vi "Clear Errors - Ext.vi"(8 "error in (no error)":errorcluster, 11 "specific error code to clear (0: all)":i32) -> (0 "error out":errorcluster)   [LabVIEW 2019]
doc: "<b>Description</b> This VI clears errors and can be used as an alternative to the stock Clear Errors VI. This VI is not not pull in any other library dependencies.\n\n<b>Inputs</b>\n<b>specific error code to clear</b>: Optionally specifies a specific error to clear.\n\n<b>Outputs</b>\n<b>error out</b>: Empty error if no specific error was specified or the specific error matches the input error.\n\nBSD 3-Clause License\n\nCopyright (c) 2021, TauTerra, LLC\nAll rights reserved.\n\nRedistribution and use in source and binary forms, with or without\nmodification, are permitted provided that the following conditions are met:\n\n1. Redistributions of source code must retain the above copyright notice, this\n list of conditions and the following disclaimer.\n\n2. Redistributions in binary form must reproduce the above copyright notice,\n this list of conditions and the following disclaimer in the documentation\n and/or other materials provided with the distribution.\n\n3. Neither the name of the copyright holder nor the names of its\n contributors may be used to endorse or promote products derived from\n this software without specific prior written permission.\n\nTHIS SOFTWARE IS PROVIDED BY THE COPYRIGHT HOLDERS AND CONTRIBUTORS \"AS IS\"\nAND ANY EXPRESS OR IMPLIED WARRANTIES, INCLUDING, BUT NOT LIMITED TO, THE\nIMPLIED WARRANTIES OF MERCHANTABILITY AND FITNESS FOR A PARTICULAR PURPOSE ARE\nDISCLAIMED. IN NO EVENT SHALL THE COPYRIGHT HOLDER OR CONTRIBUTORS BE LIABLE\nFOR ANY DIRECT, INDIRECT, INCIDENTAL, SPECIAL, EXEMPLARY, OR CONSEQUENTIAL\nDAMAGES (INCLUDING, BUT NOT LIMITED TO, PROCUREMENT OF SUBSTITUTE GOODS OR\nSERVICES; LOSS OF USE, DATA, OR PROFITS; OR BUSINESS INTERRUPTION) HOWEVER\nCAUSED AND ON ANY THEORY OF LIABILITY, WHETHER IN CONTRACT, STRICT LIABILITY,\nOR TORT (INCLUDING NEGLIGENCE OR OTHERWISE) ARISING IN ANY WAY OUT OF THE USE\nOF THIS SOFTWARE, EVEN IF ADVISED OF THE POSSIBILITY OF SUCH DAMAGE."
panel:
  out "specific error cleared?":bool
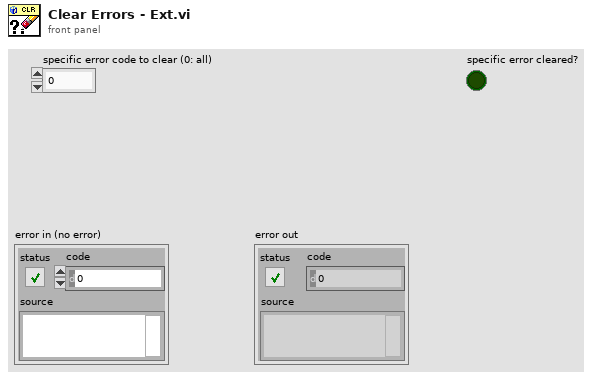
[diagram p1: front panel]
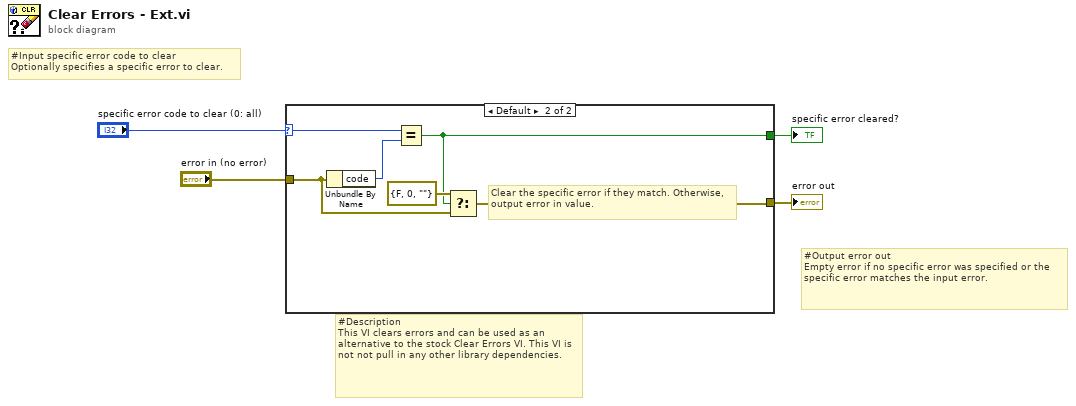
[diagram p0: block diagram]
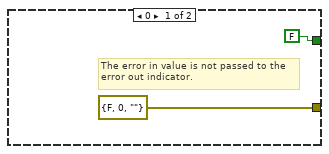
[diagram p2: hidden frame]
diagram:
  # "#Output error out\nEmpty error if no specific error was specified or the specific error matches the input error."
  # "#Input specific error code to clear\nOptionally specifies a specific error to clear."
  # "#Description\nThis VI clears errors and can be used as an alternative to the stock Clear Errors VI. This VI is not not pull in any other library dependencies."
  n1 = case shown="Default" "specific error code to clear (0: all)" {
    selector: "specific error code to clear (0: all)" -> [_ w11]
    tunnel: "error in (no error)" -> [_ w10]
    tunnel: [errorcluster {"status"=FALSE, "code"=0, "source"=""} ("error constant") w7] -> w1
    tunnel: [FALSE w8] -> w3
    frame 0 {
      # "The error in value is not passed to the\nerror out indicator."
    }
    frame Default {
      # "Clear the specific error if they match. Otherwise, output error in value."
      n2 = Unbundle By Name(w10) -> ("code"=w12:i32)
      n3 = Equal?(x=w11, y=w12) -> (x = y?=w8:bool)
      n4 = Select(t=errorcluster {"status"=FALSE, "code"=0, "source"=""} ("error constant"), s=w8, f=w10) -> (s? t:f=w7:errorcluster)
    }
  }
  "error out" <- w1
  "specific error cleared?" <- w3
